vi "Display Information.vi"(8 "error in (no error)":errorcluster, 11 "Master in":refnum<class "MASTER.lvclass">) -> (0 "error out":errorcluster, 1 "Passwords":string[](array[string]), 3 "Master out":refnum<class "MASTER.lvclass">, 4 "Recipe Indicator":string[][](array[string]), 7 "Dryer Controls":T1)   [LabVIEW 2014, in "Files Library.lvlib" / "Master.lvclass"]
uses:
  MASTER/MASTER.lvclass
  MASTER/MASTER.lvclass/MASTER.ctl
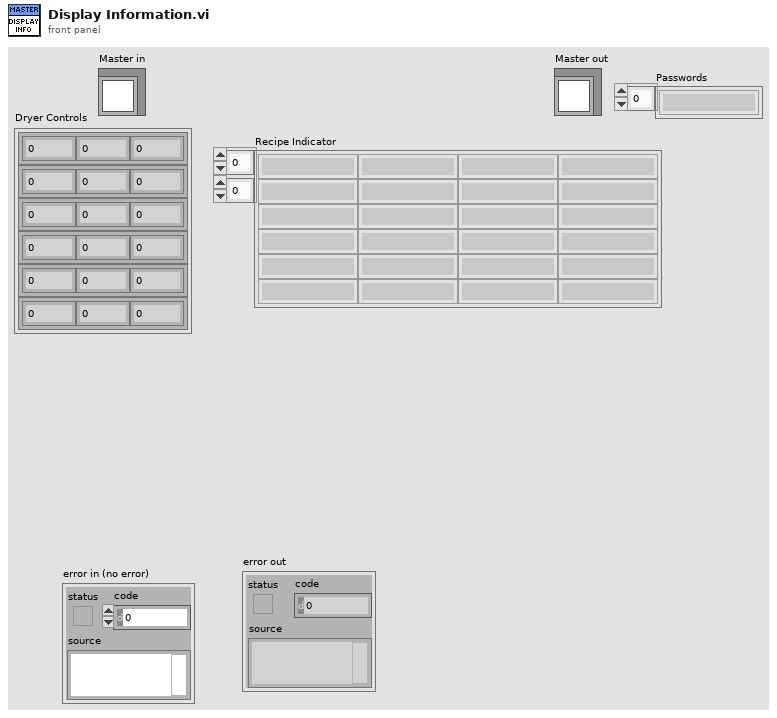
[diagram p1: front panel]
types:
  T1 = cluster{"Dryer Controls":cluster{"speed":u16, "Temp":u16, " Time":u16}, "Dryer Controls 2":cluster{"speed":u16, "Temp":u16, " Time":u16}, "Dryer Controls 3":cluster{"speed":u16, "Temp":u16, " Time":u16}, "Dryer Controls 4":cluster{"speed":u16, "Temp":u16, " Time":u16}, "Dryer Controls 5":cluster{"speed":u16, "Temp":u16, " Time":u16}, "Dryer Controls 6":cluster{"speed":u16, "Temp":u16, " Time":u16}}
  T2 = typedef "Recipes Indicators.ctl" = cluster{"Speed":string, "Temperature SP":string, "Time Limit":string, "Direction":string}
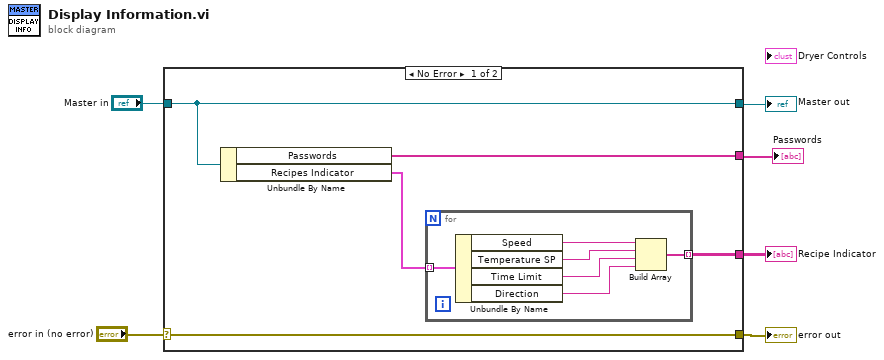
[diagram p0: block diagram]
diagram:
  n1 = case shown="No Error" "error in (no error)" {
    selector: "error in (no error)" -> [w11 w18]
    tunnel: [w11 w18] -> w5
    tunnel: [w10 w19] -> w3
    tunnel: "Master in" -> [w10 w19]
    tunnel: [w9 _] -> w2
    tunnel: [w7 _] -> w1
    frame No Error {
      n2 = Unbundle By Name(w10) -> ("Passwords"=w9:string[], "Recipes Indicator"=w8:T2[])
      n3 = for {
        tunnel: w8 -> [w17] mode=indexing
        tunnel: [w12] -> w7 mode=indexing
        n4 = Unbundle By Name(w17) -> ("Speed"=w16:string, "Temperature SP"=w15:string, "Time Limit"=w14:string, "Direction"=w13:string)
        n5 = Build Array(w16, w15, w14, w13) -> (w12:string[])
      }
    }
    frame Error {
    }
  }
  "error out" <- w5
  "Master out" <- w3
  "Recipe Indicator" <- w1
  "Passwords" <- w2
